vi "test_replace named format specifier.vi"(7 "format string":string="%{str}$s\n%{dbl}$x\n%{dbl}$o\n%{dbl}$b\n%{dbl}$d\n%{dbl}$u\n%{dbl}$f\n%{dbl}$e\n%{dbl}$g\n%{dbl}$p\n%{path}$s\n%{i32}$d\n%{timestamp}$T\n%{enum}$s\n%{enum}$d\n%{sub.quote}$s\n%{sub.val}$f", 8 "error in":errorcluster, 11 "data":T1={"str"="hello, world", "dbl"=-420.69, "path"=path "path/to/nowhere", "i32"=123645789, "timestamp"=timestamp(3820544415.5264506 s since 1904-01-01), "enum"=enum."third", "sub"={"quote"="good to be here", "val"=1589624.0}, "name.with.dots"=15987, "name\\with\\slashes"=7862199, "name.with\\both"=16874654}) -> (0 "error out":errorcluster, 3 "resulting string":string="hello, world\nFFFFFFFFFFFFFE5B\n1777777777777777777133\n1111111111111111111111111111111111111111111111111111111001011011\n-421\n0\n-420.690000\n-4.206900E+2\n-420.690000\n-420.690000\npath\\to\\nowhere\n123645789\n10:20:15.526 PM 1/23/2025\nthird\n2\ngood to be here\n1589624.000000")   [LabVIEW 2018]
uses:
  api/configuration/formatters/format_string_formatter/Format String.lvclass
panel:
  # "Connector Pane"
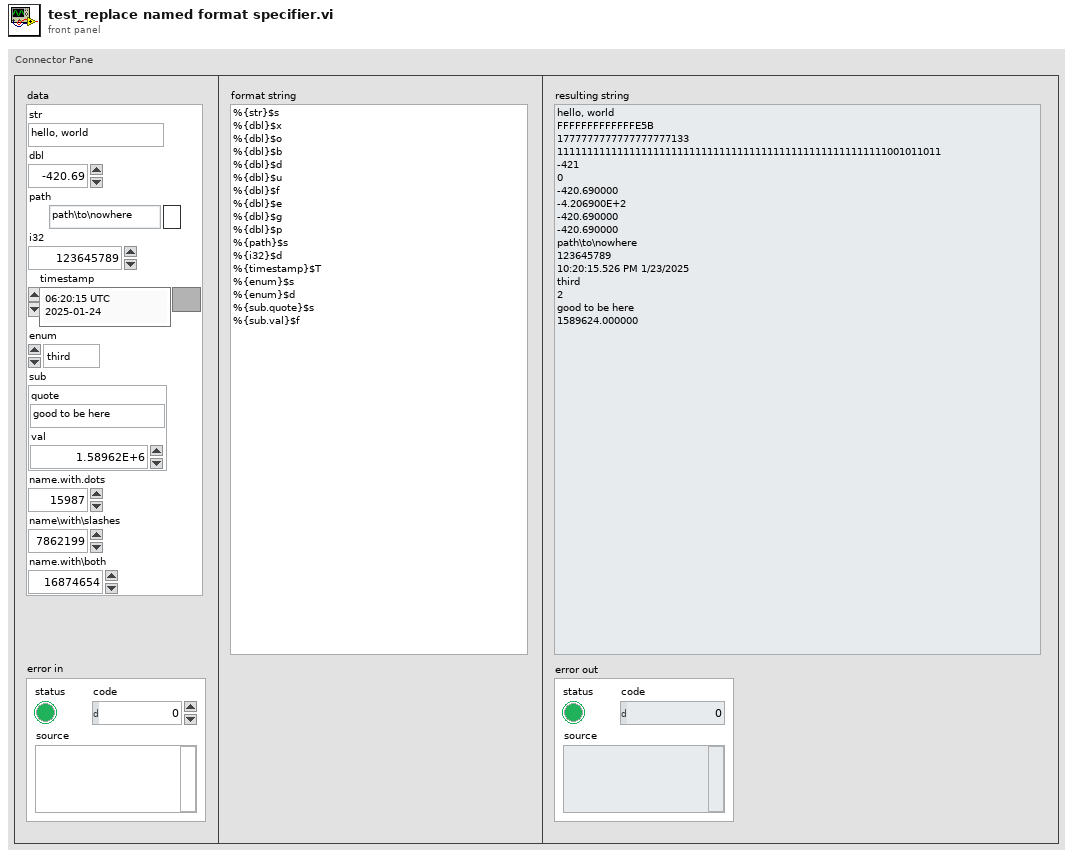
[diagram p1: front panel]
types:
  T1 = cluster{"str":string, "dbl":dbl, "path":path, "i32":i32, "timestamp":timestamp, "enum":enum16{"first", "second", "third"}, "sub":cluster{"quote":string, "val":dbl}, "name.with.dots":i32, "name\\with\\slashes":i32, "name.with\\both":i32}
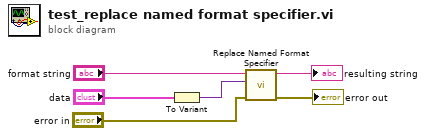
[diagram p0: block diagram]
diagram:
  n1 = To Variant(anything="data") -> (Variant=w5:variant)
  n2 = call "Replace Named Format Specifier.vi"("error in (no error)"="error in", "data"=w5, "format string"="format string") -> ("error out"=→"error out":errorcluster, "resulting string"=→"resulting string":string)  [unwired: 7 in]
